vi "motorPwm.vi"(7 "reverse?":bool, 8 "error in (no error)":errorcluster, 10 "Speed (PWM)":dbl) -> (0 "error out":errorcluster)   [LabVIEW 2019, in "SJCube.lvlib"]
uses:
  SJCube.lvlib
  KNRm_ReMi_OS6.lvlibp/KNRm_ReMi_Toolkit/Control/MotorNumberSelect.ctl
  <vilib>/myRIO/Common/Instrument Driver Framework/Utilities/typedefs/myRIO Generic Hardware Reference.ctl
  <vilib>/myRIO/Common/Instrument Driver Framework/Utilities/typedefs/myRIO v1.0 Reference.ctl
  <vilib>/myRIO/Common/Instrument Driver Framework/Utilities/typedefs/Generic FPGA Reference.ctl
  <vilib>/myRIO/Common/Instrument Driver Framework/Utilities/typedefs/Hardware Version Enum.ctl
  <vilib>/userDefined/High Color/nirio_resource_hc.ctl
  <vilib>/myRIO/Common/Instrument Driver Framework/Utilities/vis/Is FPGA Ref Available.vi
  <vilib>/myRIO/Instrument Drivers/Onboard IO/PWM/typedefs/PWM Configuration.ctl
  <vilib>/myRIO/Instrument Drivers/Onboard IO/PWM/PWM.lvlib
  <vilib>/myRIO/Common/Instrument Driver Framework/myRIO v1.0/PWM/typedefs/PWM Channels Enum.ctl
  <vilib>/myRIO/Instrument Drivers/Onboard IO/PWM/typedefs/PWM Reference.ctl
  <vilib>/myRIO/Instrument Drivers/Onboard IO/PWM/vis/Set Duty Cycle and Frequency.vi
  <vilib>/myRIO/Instrument Drivers/Onboard IO/PWM/vis/myRIO PWM Open.xnode
  <vilib>/myRIO/Express VI/Onboard IO/PWM/PWM Express VI.xnode
  <vilib>/myRIO/Common/Instrument Driver Framework/myRIO v1.0/DIO/typedefs/DIO Channels Enum.ctl
  <vilib>/myRIO/Common/Instrument Driver Framework/myRIO v1.0/DIO/typedefs/DIO Channels List.ctl
  <vilib>/myRIO/Instrument Drivers/Onboard IO/DIO/typedefs/DIO Reference.ctl
  <vilib>/myRIO/Instrument Drivers/Onboard IO/DIO/DIO.lvlib
  <vilib>/myRIO/Instrument Drivers/Onboard IO/DIO/vis/Write.vi
  <vilib>/myRIO/Instrument Drivers/Onboard IO/DIO/vis/myRIO DIO Open.xnode
  <vilib>/myRIO/Express VI/Onboard IO/DO/DO Express VI.xnode
  <vilib>/myRIO/Common/Instrument Driver Framework/myRIO v1.0/DIO/vis/myRIO v1.2 Open DIO.vi
  <vilib>/myRIO/Common/Instrument Driver Framework/myRIO v1.0/PWM/vis/myRIO v1.2 Open PWM.vi
  KNRm_ReMi_OS6.lvlibp
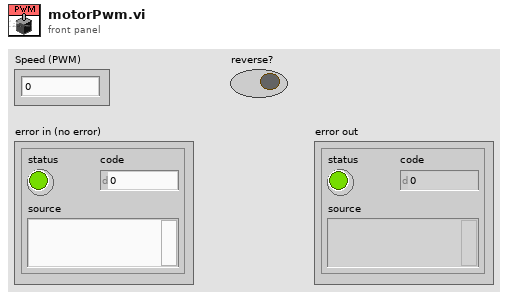
[diagram p1: front panel]
types:
  T1 = typedef "DIO.lvlib/DIO Reference.ctl" = cluster{"myRIO Reference":T2, "DIO Channels List":T6}
  T2 = typedef "myRIO Generic Hardware Reference.ctl" = cluster{"myRIO Model":T3, "myRIO Hardware Reference":T4}
  T3 = typedef "Hardware Version Enum.ctl" = enum16{"Unknown", "myRIO-1900", "myRIO-1950", "roboRIO", "NI ELVIS RIO CM", "ELVIS III"}
  T4 = typedef "myRIO v1.0 Reference.ctl" = cluster{"Generic FPGA Reference":T5, "Allow multiple opens":bool}
  T5 = typedef "Generic FPGA Reference.ctl" = refnum<k20>
  T6 = typedef "DIO Channels List.ctl" = T7[]
  T7 = typedef "DIO Channels Enum.ctl" = enum16{"Not Connected", "C/DIO0", "C/DIO1", "C/DIO2", "C/DIO3", "C/DIO4", "C/DIO5", "C/DIO6", "C/DIO7", "A/DIO0", "A/DIO1", "A/DIO2", "A/DIO3", "A/DIO4", "A/DIO5", "A/DIO6", "A/DIO7", "A/DIO8", "A/DIO9", "A/DIO10", "A/DIO11", "A/DIO12", "A/DIO13", "A/DIO14", "A/DIO15", "A/DIO16", "A/DIO17", "A/DIO18", "A/DIO19", "B/DIO0", "B/DIO1", "B/DIO2", "B/DIO3", "B/DIO4", "B/DIO5", "B/DIO6", "B/DIO7", "B/DIO8", "B/DIO9", "B/DIO10", "B/DIO11", "B/DIO12", "B/DIO13", "B/DIO14", "B/DIO15", "B/DIO16", "B/DIO17", "B/DIO18", "B/DIO19", "LED0", "LED1", "LED2", "LED3", "Button0", "DIO/DIO0", "DIO/DIO1", "DIO/DIO2", "DIO/DIO3", "DIO/DIO4", "DIO/DIO5", "DIO/DIO6", "DIO/DIO7", "DIO/DIO8", "DIO/DIO9", "SPI/CS0", "SPI/CS1", "SPI/CS2", "SPI/CS3", "LED RADIO (Green)", "LED RADIO (Red)", "LED COMM (Green)", "LED COMM (Red)", "LED MODE (Green)", "LED MODE (Red)"}
  T8 = typedef "nirio_resource_hc.ctl" = tag
  T9 = typedef "PWM.lvlib/PWM Reference.ctl" = cluster{"myRIO Reference":T2, "PWM Channels Enum":T10, "PWM Configuration":T11}
  T10 = typedef "PWM Channels Enum.ctl" = enum16{"Not Connected", "C/PWM0", "C/PWM1", "A/PWM0", "A/PWM1", "A/PWM2", "A/PWM3", "A/PWM4", "A/PWM5", "A/PWM6", "A/PWM7", "A/PWM8", "A/PWM9", "A/PWM10", "A/PWM11", "A/PWM12", "A/PWM13", "A/PWM14", "A/PWM15", "A/PWM16", "A/PWM17", "A/PWM18", "A/PWM19", "B/PWM0", "B/PWM1", "B/PWM2", "B/PWM3", "B/PWM4", "B/PWM5", "B/PWM6", "B/PWM7", "B/PWM8", "B/PWM9", "B/PWM10", "B/PWM11", "B/PWM12", "B/PWM13", "B/PWM14", "B/PWM15", "B/PWM16", "B/PWM17", "B/PWM18", "B/PWM19", "PWM/PWM0", "PWM/PWM1", "PWM/PWM2", "PWM/PWM3", "PWM/PWM4", "PWM/PWM5", "PWM/PWM6", "PWM/PWM7", "PWM/PWM8", "PWM/PWM9"}
  T11 = typedef "PWM.lvlib/PWM Configuration.ctl" = cluster{"Frequency":dbl, "Duty Cycle":dbl}
  T12 = typedef "KNRm_ReMi_OS6.lvlibp/MotorNumberSelect.ctl" = enum16{"DS1", "DS2", "DS3", "DS4"}
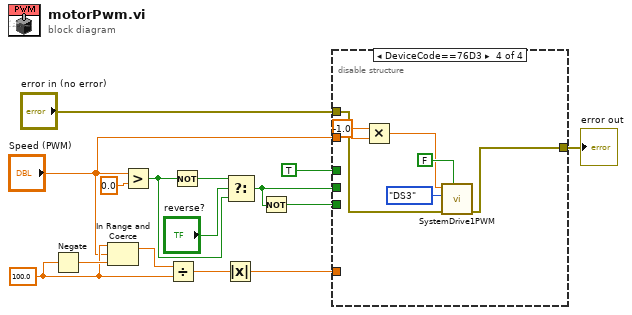
[diagram p0: block diagram]
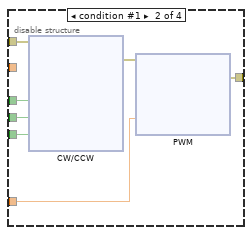
[diagram p3: hidden frame]
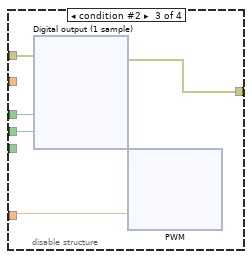
[diagram p4: hidden frame]
diagram:
  w13 = 100.0 ("upper limit")
  n1 = Negate(x=w13) -> (-x=w14:dbl)
  n2 = In Range and Coerce(upper limit=w13, x="Speed (PWM)", lower limit=w14) -> (coerced(x)=w15:dbl)  [unwired: 1 out]
  n3 = Greater?(x="Speed (PWM)", y=0.0) -> (0:w3:bool)
  n4 = Divide(x=w15, y=w13) -> (x/y=w12:dbl)
  n5 = Not(x=w3) -> (.not. x?=w4:bool)
  n6 = Absolute Value(x=w12) -> (abs(x)=w11:dbl)
  n7 = Select(t=w4, s="reverse?", f=w3) -> (s? t:f=w2:bool)
  n8 = Not(x=w2) -> (.not. x?=w7:bool)
  n9 = disable-structure shown="DeviceCode==76D3" {
    disable-tunnel: w11 -> [_ w16 w95 _]
    disable-tunnel: "error in (no error)" -> [_ w21 w99 w176]
    disable-tunnel: [_ w20 w96 w175] -> w8
    disable-tunnel: w7 -> [_ w17 _ _]
    disable-tunnel: TRUE ("EN (A/DIO5)") -> [_ w19 w98 _]
    disable-tunnel: w2 -> [_ w18 w97 _]
    disable-tunnel: "Speed (PWM)" -> [_ _ _ w173]
    frame condition #0 {
    }
    frame condition #1 {
      n10 = xnode "CW/CCW"("EN (A/DIO5)"=w19, "INA (A/DIO6)"=w18, "INB (A/DIO7)"=w17, "error in (no error)"=w21) -> ("error out"=w22:errorcluster)
      n11 = xnode "PWM"("Duty Cycle"=w16, "error in (no error)"=w22) -> ("error out"=w20:errorcluster)
    }
    frame condition #2 {
      n12 = xnode ("Digital output (1 sample)")("A/DIO0 (Pin 11)"=w98, "A/DIO1 (Pin 13)"=w97, "error in (no error)"=w99) -> ("error out"=w96:errorcluster)
      n13 = xnode ("PWM")("Duty Cycle"=w95) -> ()  [unwired: 1 in, 1 out]
    }
    frame condition #3 (active) {
      n14 = Multiply(x=-1.0, y=w173) -> (x*y=w172:dbl)
      n15 = call "SystemDrive1PWM.vi"("Reset"=FALSE, "error in"=w176, "MotorNumberSelect"=MotorNumberSelect."DS3", "MotorSpeed(PWM%)"=w172) -> ("error out"=w175:errorcluster)  [unwired: 6 in, 1 out]
    }
  }
  "error out" <- w8
